vi "Get Light Intensity Voltage Source.vi"(8 "error in (no error)":errorcluster, 11 "Gantry in":refnum<class "Gantry.lvclass">) -> (0 "error out":errorcluster, 2 "Source Type":string, 3 "Gantry out":refnum<class "Gantry.lvclass">)   [LabVIEW 2017, in "Gantry.lvclass"]
uses:
  Gantry.lvclass
  FlexWorktable/FlexWorktable.lvclass
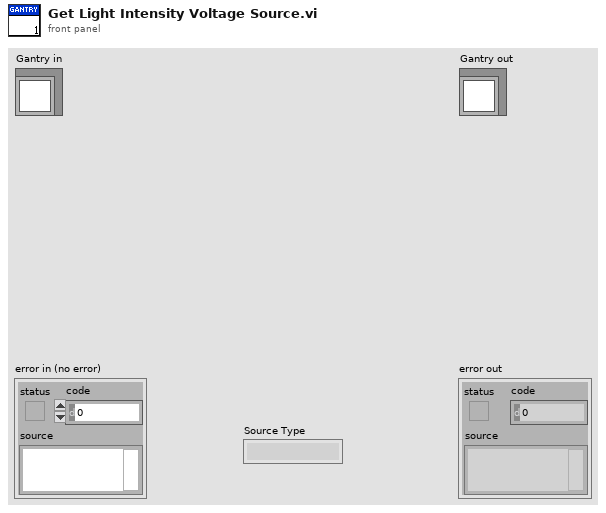
[diagram p1: front panel]
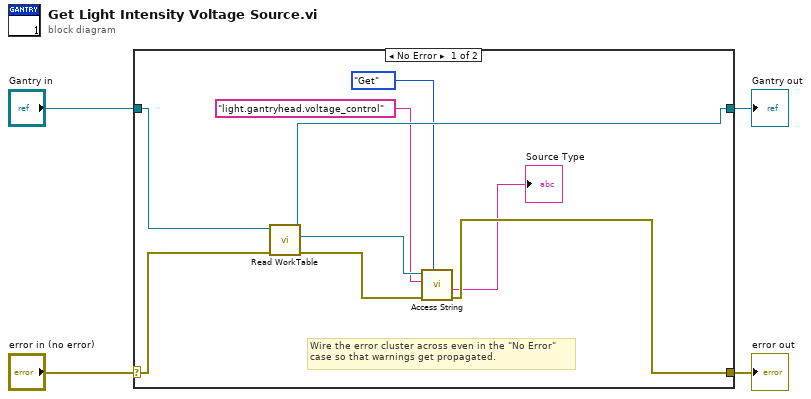
[diagram p0: block diagram]
diagram:
  n1 = case shown="No Error" "error in (no error)" {
    selector: "error in (no error)" -> [w8 w15]
    tunnel: [w6 w15] -> w3
    tunnel: [w12 w14] -> w1
    tunnel: "Gantry in" -> [w13 w14]
    frame No Error {
      # "Wire the error cluster across even in the \"No Error\"\ncase so that warnings get propagated."
      n2 = call-dynamic "Read WorkTable.vi"("error in"=w8, "Gantry Class in"=w13) -> ("error out"=w7:errorcluster, "Worktable"=w11:refnum<class "FlexWorktable.lvclass">, "Gantry Class out"=w12:refnum<class "Gantry.lvclass">)  [unwired: 7 in]
      n3 = call-dynamic "Access String.vi"("Get/Set"=enum16{"Get", "Set"}."Get", "error in (no error)"=w7, "Key"="light.gantryhead.voltage_control", "FlexWorktable in"=w11) -> ("error out"=w6:errorcluster, "Value out"=→"Source Type":string)  [unwired: 5 in, 1 out]
    }
    frame Error {
    }
  }
  "error out" <- w3
  "Gantry out" <- w1
